vi "624 Fast Talon Set Reference.vi"(8 "error in (no error)":errorcluster, 10 "Feedback Reference":T8, 11 "MotorControlDevRef":T1={"DeviceStatus"={"status"=FALSE, "code"=0, "source"=""}, "Type"=enum."PWM", "PWM"={"PWM Channel"=enum."Invalid", "DeadBand"={"Name"="", "maxPositivePwm"=0, "minPositivePwm"=0, "centerPwm"=0, "maxNegativePwm"=0, "minNegativePwm"=0, "angularRange"=0}}, "CAN"={"Device Number"=0, "Control Mode"=enum."Percent VBus", "Semaphore"=refnum, "Max Vout"=12.0, "TalonSRX Control Mode"=enum."Percent VBus"}, "Invert"=FALSE}) -> (0 "error Out":errorcluster, 3 "MotorControlDevRef Out":T1={"DeviceStatus"={"status"=FALSE, "code"=0, "source"=""}, "Type"=enum."PWM", "PWM"={"PWM Channel"=enum."Invalid", "DeadBand"={"Name"="", "maxPositivePwm"=0, "minPositivePwm"=0, "centerPwm"=0, "maxNegativePwm"=0, "minNegativePwm"=0, "angularRange"=0}}, "CAN"={"Device Number"=0, "Control Mode"=enum."Percent VBus", "Semaphore"=refnum, "Max Vout"=12.0, "TalonSRX Control Mode"=enum."Percent VBus"}, "Invert"=FALSE})   [LabVIEW 2015]
uses:
  <vilib>/Rock Robotics/WPI/MotorControl/WPI_MotorControlDeviceRef.ctl
  <vilib>/Rock Robotics/WPI/MotorControl/WPI_MotorControlType.ctl
  <vilib>/Rock Robotics/SystemInterfaces/DIO/FPGA_DIOPWMChannel.ctl
  <vilib>/Rock Robotics/WPI/PWM/WPI_PWMDeadband.ctl
  <vilib>/Rock Robotics/WPI/CAN/Jaguar/SubVIs/WPI_CANJaguar_ControlMode.ctl
  <vilib>/Rock Robotics/WPI/CAN/TalonSRX/WPI_CANTalonSRX_APIControlMode.ctl
  <vilib>/Rock Robotics/WPI/CAN/TalonSRX/WPI_CANTalonSRX_APIFeedbackSelect.ctl
  <vilib>/Rock Robotics/WPI/CAN/TalonSRX/WPI_CANTalonSRX_GlobalOps.ctl
  <vilib>/Rock Robotics/WPI/CAN/TalonSRX/WPI_CANTalonSRX_FeedbackSelect.ctl
  Common Code/Change Detect Boolean.vi
  Common Code/Change Detect Int.vi
panel:
  in  "Reverse Feedback":bool
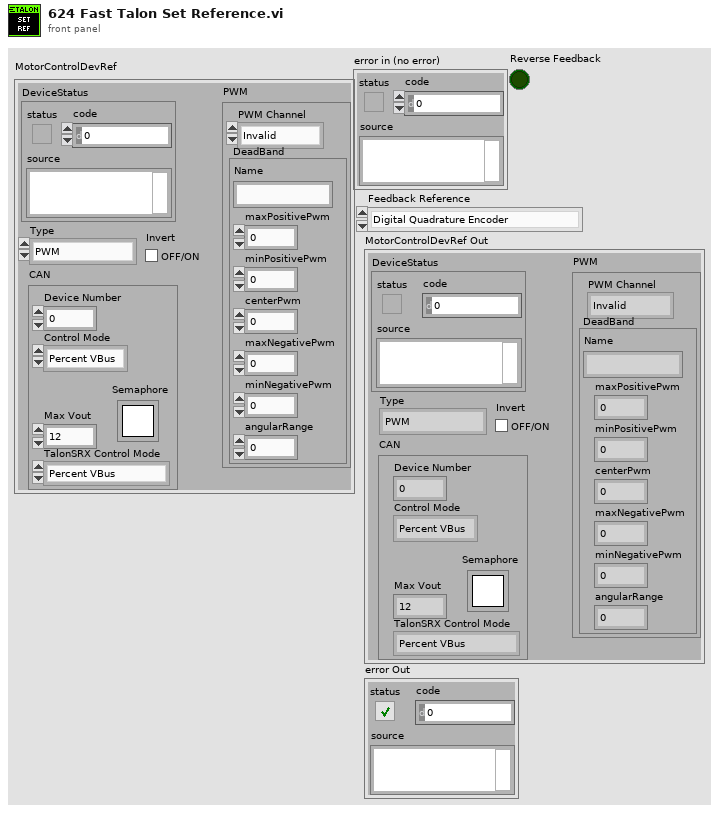
[diagram p1: front panel]
types:
  T1 = typedef "WPI_MotorControlDeviceRef.ctl" = cluster{"DeviceStatus":errorcluster, "Type":T2, "PWM":cluster{"PWM Channel":T3, "DeadBand":T4}, "CAN":cluster{"Device Number":u8, "Control Mode":T5, "Semaphore":T6, "Max Vout":dbl, "TalonSRX Control Mode":T7}, "Invert":bool}
  T2 = typedef "WPI_MotorControlType.ctl" = enum16{"PWM", "CAN", "CANTalonSRX"}
  T3 = typedef "FPGA_DIOPWMChannel.ctl" = enum8{"PWM 0", "PWM 1", "PWM 2", "PWM 3", "PWM 4", "PWM 5", "PWM 6", "PWM 7", "PWM 8", "PWM 9", "PWM MXP 0", "PWM MXP 1", "PWM MXP 2", "PWM MXP 3", "PWM MXP 4", "PWM MXP 5", "PWM MXP 6", "PWM MXP 7", "PWM MXP 8", "PWM MXP 9", "Invalid"}
  T4 = typedef "WPI_PWMDeadband.ctl" = cluster{"Name":string, "maxPositivePwm":i32, "minPositivePwm":i32, "centerPwm":i32, "maxNegativePwm":i32, "minNegativePwm":i32, "angularRange":u16}
  T5 = typedef "WPI_CANJaguar_ControlMode.ctl" = enum8{"Percent VBus", "Current", "Speed", "Position", "Voltage"}
  T6 = typedef "Semaphore RefNum" = refnum<k1>
  T7 = typedef "WPI_CANTalonSRX_APIControlMode.ctl" = enum8{"Percent VBus", "Speed", "Position", "Slave", "Unchanged / Invalid", "Voltage Compensation", "Current", "Motion Profile"}
  T8 = typedef "WPI_CANTalonSRX_APIFeedbackSelect.ctl" = enum16{"Digital Quadrature Encoder", "Analog Potentiometer", "Analog Encoder", "Count on Quad-A (Rising-Edge)", "Count on Quad-A (Falling-Edge)", "CTR Magnetic Enc (Absolute)", "CTR Magnetic Enc (Relative)", "Pulse Width"}
  T9 = typedef "WPI_CANTalonSRX_GlobalOps.ctl" = enum16{"Read For Send", "Write After Receive General", "Write After Receive Feedback", "Write After Receive Encoder", "Write After Receive Ain", "Write Error", "Get All", "Set Output", "Set Mode", "Set Master ID", "Set Brake Mode", "Set Reverse Feedback Sensor", "Set Reverse Closed Loop Output", "Set Override Limits", "Set Forward Limit Enabled", "Set Reverse Limit Enabled", "Set Feedback Select", "Set Profile Select", "Set Throttle Ramp Rate", "Disable", "Set Enc Codes Per Rev", "Set Num Pot Turns", "Set Control Frame Rate", "Enable Legacy Control", "Write After Receive Pulse Width", "Set Enable Frame Rate", "Write After Receive Motion Profile", "Set Motion Profile Flow Control", "Set Motion Profile Control Frame Rate"}
  T10 = typedef "WPI_CANTalonSRX_FeedbackSelect.ctl" = u8
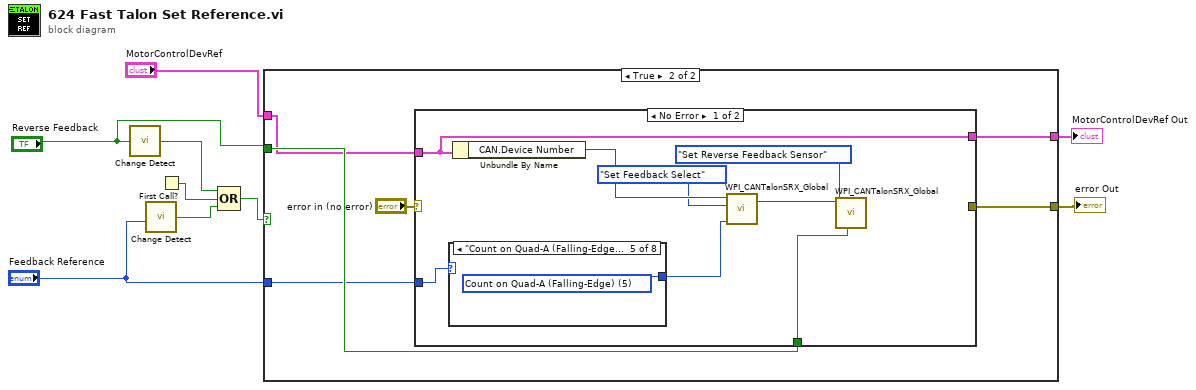
[diagram p0: block diagram]
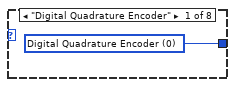
[diagram p3: hidden frame]
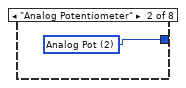
[diagram p4: hidden frame]
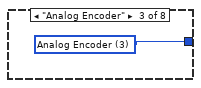
[diagram p5: hidden frame]
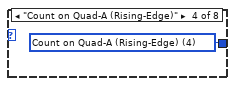
[diagram p6: hidden frame]
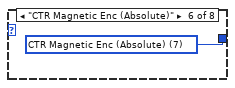
[diagram p7: hidden frame]
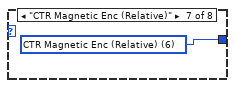
[diagram p8: hidden frame]
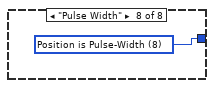
[diagram p9: hidden frame]
diagram:
  n1 = call-poly "Change Detect.vi"("In"="Reverse Feedback") -> ("Changed?"=w2:bool)
  n2 = call-poly "Change Detect.vi"("In"="Feedback Reference") -> ("Changed?"=w6:bool)
  n3 = First Call?() -> (First Call?: T/F=w5:bool)
  n4 = Compound Arithmetic op=OR(w2, w5, w6) -> (w4:bool)
  n5 = case shown="True" w4 {
    tunnel: "Reverse Feedback" -> [_ w15]
    tunnel: [w10 w14] -> w9
    tunnel: [_ w13] -> w8
    tunnel: "Feedback Reference" -> [_ w12]
    tunnel: "MotorControlDevRef" -> [w10 w11]
    frame False {
    }
    frame True {
      n6 = case shown="No Error" "error in (no error)" {
        selector: "error in (no error)" -> [_ w33]
        tunnel: w11 -> [w23 w34]
        tunnel: w12 -> [w24 _]
        tunnel: w15 -> [w17 _]
        tunnel: [w23 w34] -> w14
        tunnel: [_ w33] -> w13
        frame No Error {
          n7 = case shown="\"Count on Quad-A (Falling-Edge)\"" w24 {
            tunnel: [w25 w26 w27 w28 w29 w30 w31 w32] -> w20
            frame "Digital Quadrature Encoder" {
              w25 = T10 0 items=["Digital Quadrature Encoder"=0, "Analog Pot"=2, "Analog Encoder"=3, "Count on Quad-A (Rising-Edge)"=4, "Count on Quad-A (Falling-Edge)"=5, "Position is Pulse-Width"=8] ("Talon SRX Feedback Select")
            }
            frame "Analog Potentiometer" {
              w26 = T10 2 items=["Digital Quadrature Encoder"=0, "Analog Pot"=2, "Analog Encoder"=3, "Count on Quad-A (Rising-Edge)"=4, "Count on Quad-A (Falling-Edge)"=5, "Position is Pulse-Width"=8] ("Talon SRX Feedback Select")
            }
            frame "Analog Encoder" {
              w27 = T10 3 items=["Digital Quadrature Encoder"=0, "Analog Pot"=2, "Analog Encoder"=3, "Count on Quad-A (Rising-Edge)"=4, "Count on Quad-A (Falling-Edge)"=5, "Position is Pulse-Width"=8] ("Talon SRX Feedback Select")
            }
            frame "Count on Quad-A (Rising-Edge)" {
              w28 = T10 4 items=["Digital Quadrature Encoder"=0, "Analog Pot"=2, "Analog Encoder"=3, "Count on Quad-A (Rising-Edge)"=4, "Count on Quad-A (Falling-Edge)"=5, "Position is Pulse-Width"=8] ("Talon SRX Feedback Select")
            }
            frame "Count on Quad-A (Falling-Edge)" {
              w29 = T10 5 items=["Digital Quadrature Encoder"=0, "Analog Pot"=2, "Analog Encoder"=3, "Count on Quad-A (Rising-Edge)"=4, "Count on Quad-A (Falling-Edge)"=5, "Position is Pulse-Width"=8] ("Talon SRX Feedback Select")
            }
            frame "CTR Magnetic Enc (Absolute)" {
              w30 = T10 7 items=["Digital Quadrature Encoder"=0, "Analog Pot"=2, "Analog Encoder"=3, "Count on Quad-A (Rising-Edge)"=4, "Count on Quad-A (Falling-Edge)"=5, "Position is Pulse-Width"=8, "CTR Magnetic Enc (Relative)"=6, "CTR Magnetic Enc (Absolute)"=7] ("Talon SRX Feedback Select")
            }
            frame "CTR Magnetic Enc (Relative)" {
              w31 = T10 6 items=["Digital Quadrature Encoder"=0, "Analog Pot"=2, "Analog Encoder"=3, "Count on Quad-A (Rising-Edge)"=4, "Count on Quad-A (Falling-Edge)"=5, "Position is Pulse-Width"=8, "CTR Magnetic Enc (Relative)"=6, "CTR Magnetic Enc (Absolute)"=7] ("Talon SRX Feedback Select")
            }
            frame "Pulse Width" {
              w32 = T10 8 items=["Digital Quadrature Encoder"=0, "Analog Pot"=2, "Analog Encoder"=3, "Count on Quad-A (Rising-Edge)"=4, "Count on Quad-A (Falling-Edge)"=5, "Position is Pulse-Width"=8] ("Talon SRX Feedback Select")
            }
          }
          n8 = Unbundle By Name(w23) -> ("CAN.Device Number"=w22:u8)
          n9 = call <vilib>:"WPI_CANTalonSRX_Global.vi"("Set Number"=w20, "Operation"=WPI_CANTalonSRX_GlobalOps."Set Feedback Select", "Device ID (0)"=w22) -> ("Device ID Out"=w19:u8)  [unwired: 6 in, 2 out]
          n10 = call <vilib>:"WPI_CANTalonSRX_Global.vi"("Set Boolean"=w17, "Operation"=WPI_CANTalonSRX_GlobalOps."Set Reverse Feedback Sensor", "Device ID (0)"=w19) -> ()  [unwired: 6 in, 3 out]
        }
        frame Error {
        }
      }
    }
  }
  "MotorControlDevRef Out" <- w9
  "error Out" <- w8
